vi "Test Open Write Close WAV.vi"(8 "error in (no error)":errorcluster) -> (0 "error out":errorcluster, 3 "Pass?":bool)   [LabVIEW 2020]
uses:
  G-Audio/Controls/Audio File Info.ctl
  G-Audio/Controls/WAV Codec Specific Info.ctl
  G-Audio/Controls/WAV Container Format.ctl
  G-Audio/Controls/WAV Data Format.ctl
  1cf1aa51-db2a-4942-9e31-322e6655b9cf.vi
  0eb3ae3f-735e-49b7-bf6e-320a239f98ff.vi
  6d22e323-49e0-417e-9a88-fd83a11302a6.vi
  <vilib>/Analysis/1siggen.llb/Ramp Pattern.vi
  <vilib>/Analysis/1siggen.llb/Ramp Pattern by Samples.vi
  1cf1aa51-db2a-4942-9e31-322e6655b9cf.vi/e3c26991-7fb0-4a70-b596-1cadc78d0dfb.vi
  1cf1aa51-db2a-4942-9e31-322e6655b9cf.vi/560838c1-3c21-4b88-a164-506af39aa71c.vi
  G-Audio/Private/Result To Error.vi
  0eb3ae3f-735e-49b7-bf6e-320a239f98ff.vi/fba40667-3e21-44fa-934c-95909d78721c.vi
  6d22e323-49e0-417e-9a88-fd83a11302a6.vi/15efb94c-0eeb-49fd-9ff3-8ea0cffaf39a.vi
  0eb3ae3f-735e-49b7-bf6e-320a239f98ff.vi/fba40667-3e21-44fa-934c-95909d78721c.vi/4b7b629c-2e91-4160-9820-a26af8f6e677.vi
  0eb3ae3f-735e-49b7-bf6e-320a239f98ff.vi/fba40667-3e21-44fa-934c-95909d78721c.vi/e7c4a249-ce38-42b4-8985-5fdb76b4ebfc.vi
  <vilib>/measure/masignal.llb/Sine Waveform.vi
  <vilib>/Utility/error.llb/Error Cluster From Error Code.vi
  G-Audio/Private/Copy Data.vi
  G-Audio/G-Audio.lvlib
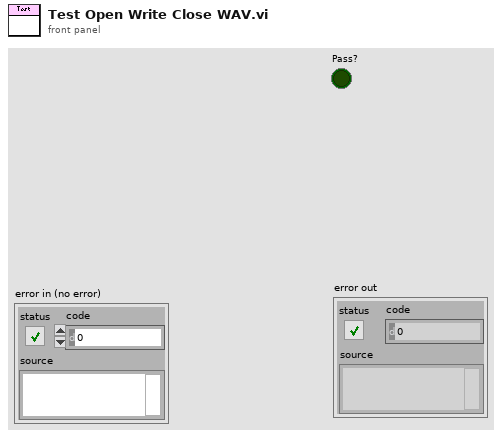
[diagram p1: front panel]
types:
  T1 = typedef "G-Audio.lvlib/WAV Codec Specific Info.ctl" = cluster{"Container Format":T2, "Data Format":T3}
  T2 = typedef "G-Audio.lvlib/WAV Container Format.ctl" = enum32{"RIFF", "Wave64"}
  T3 = typedef "G-Audio.lvlib/WAV Data Format.ctl" = u32
  T4 = typedef "G-Audio.lvlib/Audio File Info.ctl" = cluster{"Sample Rate (Hz)":u32, "Channels":u32, "Bit Depth":u32}
  T5 = typedef "G-Audio.lvlib/Audio File Refnum.ctl" = refnum<file>
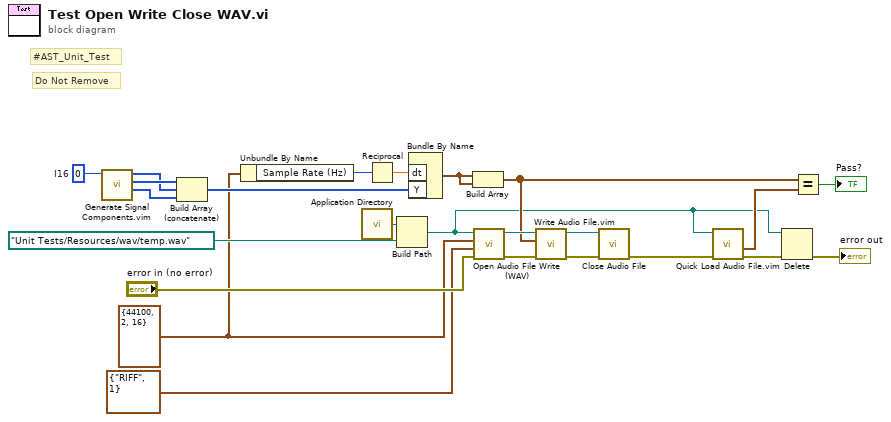
[diagram p0: block diagram]
diagram:
  w16 = i16 0  # I16
  w2 = T4 {"Sample Rate (Hz)"=44100, "Channels"=2, "Bit Depth"=16} ("Audio File Info")
  # "Do Not Remove"
  # "#AST_Unit_Test"
  n1 = call "Generate Signal Components.vim"("Data Type"=w16) -> ("Ramp Down"=w19:i16[], "Ramp Up"=w21:i16[], "Signal"=w20:i16[])  [unwired: 8 in]
  n2 = Build Array (concatenate)(w21, w20, w19) -> (w18:i16[])
  n3 = Unbundle By Name(w2) -> ("Sample Rate (Hz)"=w4:u32)
  n4 = call <vilib>:"Application Directory.vi"() -> ("Application Directory"=w24:path)
  n5 = Reciprocal(x=w4) -> (1/x=w3:dbl)
  n6 = Build Path(base path=w24, name or relative path=path "Unit Tests/Resources/wav/temp.wav" ("Path")) -> (appended path=w7:path)
  n7 = Bundle By Name("dt"=w3, "Y"=w18) -> (w17:waveform(i16))  [unwired: 1 in]
  n8 = Build Array(w17, w17) -> (w10:waveform(i16)[])
  n9 = call "Open Audio File Write (WAV).vi"("error in (no error)"="error in (no error)", "Codec Specific Info"=T1 {"Container Format"=enum."RIFF", "Data Format"=1} ("WAV File Info"), "Audio File Info"=w2, "Path"=w7) -> ("error out"=w14:errorcluster, "Audio File Refnum"=w22:T5)  [unwired: 6 in]
  n10 = call "Write Audio File.vim"("error in (no error)"=w14, "Audio Data"=w10, "Audio File Refnum In"=w22) -> ("error out"=w13:errorcluster, "Audio File Refnum Out"=w15:T5)  [unwired: 7 in]
  n11 = call "Close Audio File.vi"("error in (no error)"=w13, "Audio File Refnum In"=w15) -> ("error out"=w11:errorcluster)  [unwired: 9 in]
  n12 = call "Quick Load Audio File.vim"("error in (no error)"=w11, "Path"=w7) -> ("error out"=w6:errorcluster, "data"=w9:waveform(i16)[])  [unwired: 4 in, 4 out]
  n13 = Delete(path (use dialog)=w7, error in=w6) -> (error out=→"error out":errorcluster)  [unwired: 3 in, 2 out]
  n14 = Equal?(x=w10, y=w9) -> (x = y?=→"Pass?":bool)
